vi "Configure Marker Frequency.vi"(8 "error in (no error)":errorcluster, 9 "Marker Frequency":dbl, 10 "Marker Number":u8=1, 11 "VNA-ZNB in":refnum<class "VNA-ZNB.lvclass">) -> (0 "error out":errorcluster, 3 "VNA-ZNB out":refnum<class "VNA-ZNB.lvclass">)   [LabVIEW 2020, in "VNA-ZNB.lvclass"]
doc: "Configure the marker frequency.\nThe marker is always set on the current active trace."
uses:
  VNA-ZNB.lvclass
  C:/Sandbox/Git_Sandbox/WiSpry Test Framework source code (LV20)/WiSpry Test Framework/Instruments/Instrument.lvclass
  Instrument.lvclass/Instrument.ctl
  Instrument.lvclass
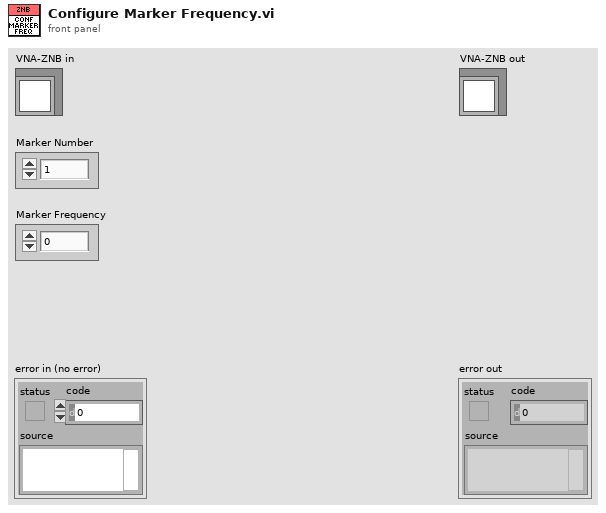
[diagram p1: front panel]
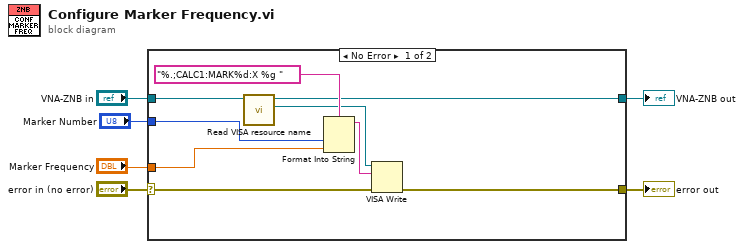
[diagram p0: block diagram]
diagram:
  n1 = case shown="No Error" "error in (no error)" {
    selector: "error in (no error)" -> [w14 w16]
    tunnel: "VNA-ZNB in" -> [w15 w17]
    tunnel: "Marker Number" -> [w12 _]
    tunnel: "Marker Frequency" -> [w11 _]
    tunnel: [w8 w16] -> w2
    tunnel: [w7 w17] -> w1
    frame No Error {
      n2 = call "Read VISA resource name.vi"("Instrument in"=w15) -> ("VISA resource name"=w10:refnum<visa-resource-name>, "Instrument out"=w7:refnum<class "VNA-ZNB.lvclass">)  [unwired: 9 in]
      n3 = Format Into String(format string="%.;CALC1:MARK%d:X %g ", w12, w11) -> (resulting string=w9:string)  [unwired: 2 in, 1 out]
      n4 = VISA Write(VISA resource name=w10, write buffer=w9, error in (no error)=w14) -> (error out=w8:errorcluster)  [unwired: 2 out]
    }
    frame Error {
    }
  }
  "error out" <- w2
  "VNA-ZNB out" <- w1
